vi "1D experiment_v119999.vi"() -> ()   [LabVIEW 2010]
uses:
  ola/Speaker Example/Action Engines/AE Access VIs/AE - Bluetooth Initialise.vi
  ola/Speaker Example/Action Engines/AE Access VIs/AE - Bluetooth Connect All.vi
  <vilib>/Utility/cursorutil.llb/Set Cursor (Cursor ID).vi
  <vilib>/Utility/file.llb/Write To Spreadsheet File (DBL).vi
  User32.dll
panel:
  out "1D Experiment":cluster{"Y":dbl[], "Y":dbl[]}[](graph) caption="Press \"Home\" in WiiMote to STOP"
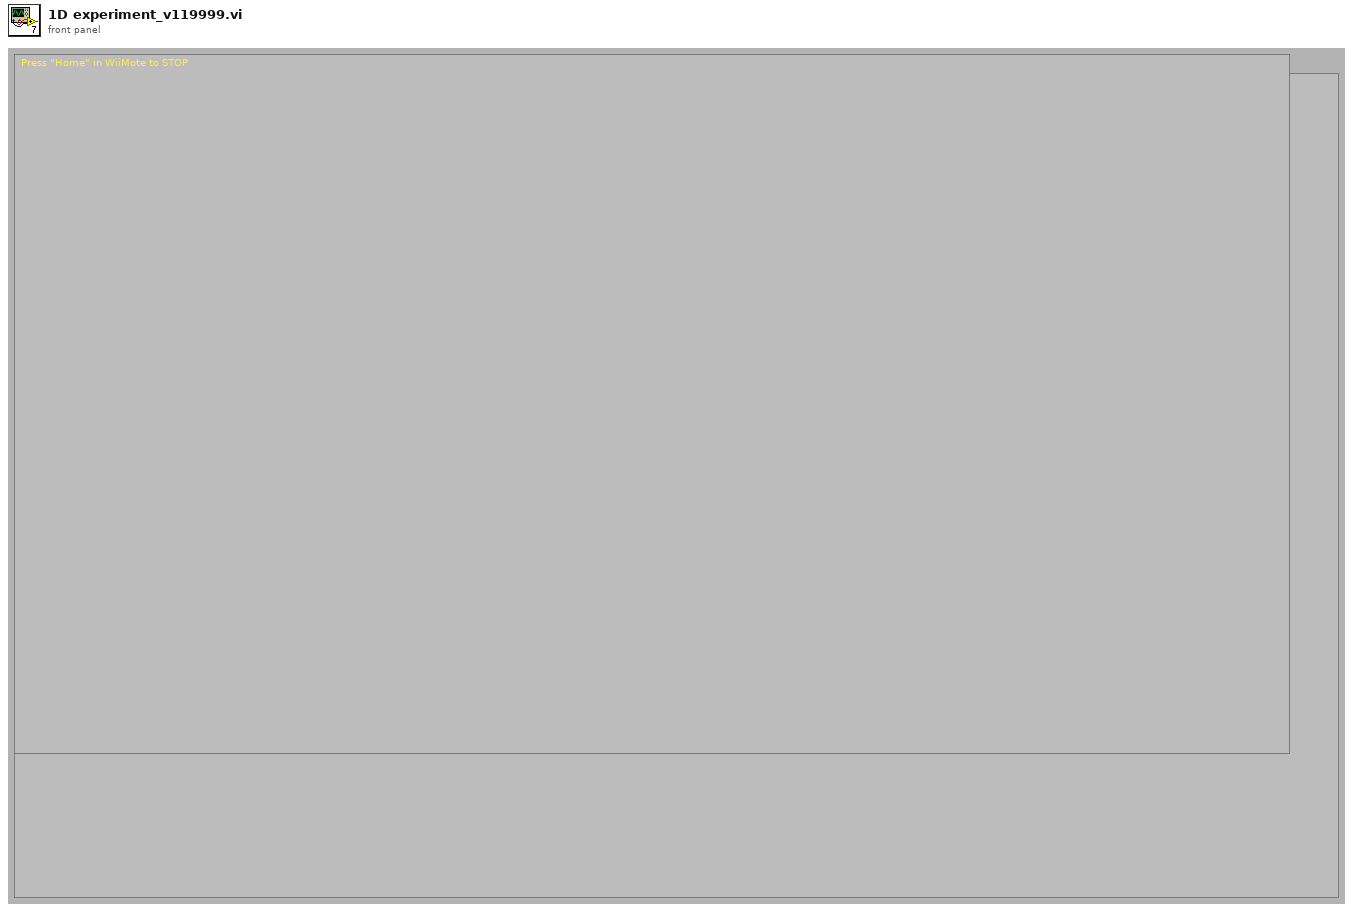
[diagram p1: front panel]
types:
  T1 = enum16{"open", "replace", "create", "open or create", "replace or create", "replace or create with confirmation"}
  T2 = cluster{"Radius":dbl, "Center":dbl, "D":dbl, "Valid":bool}
  T3 = typedef "LVAllMonitorsDisplayTypeDef.ctl" = cluster{"Bounds":cluster{"Left":i16, "Top":i16, "Right":i16, "Bottom":i16}, "Depth":i16}[]
  T4 = cluster{"Bounds":cluster{"Left":i16, "Top":i16, "Right":i16, "Bottom":i16}, "Depth":i16}
  T5 = cluster{"Left":i16, "Top":i16, "Right":i16, "Bottom":i16}
  T6 = typedef "LVPoint32TypeDef.ctl" = cluster{"Horizontal":i32, "Vertical":i32}
  T7 = cluster{"Cursor.Cursor Position:Cursor X":dbl, "Cursor.Cursor Position:Cursor X":dbl}
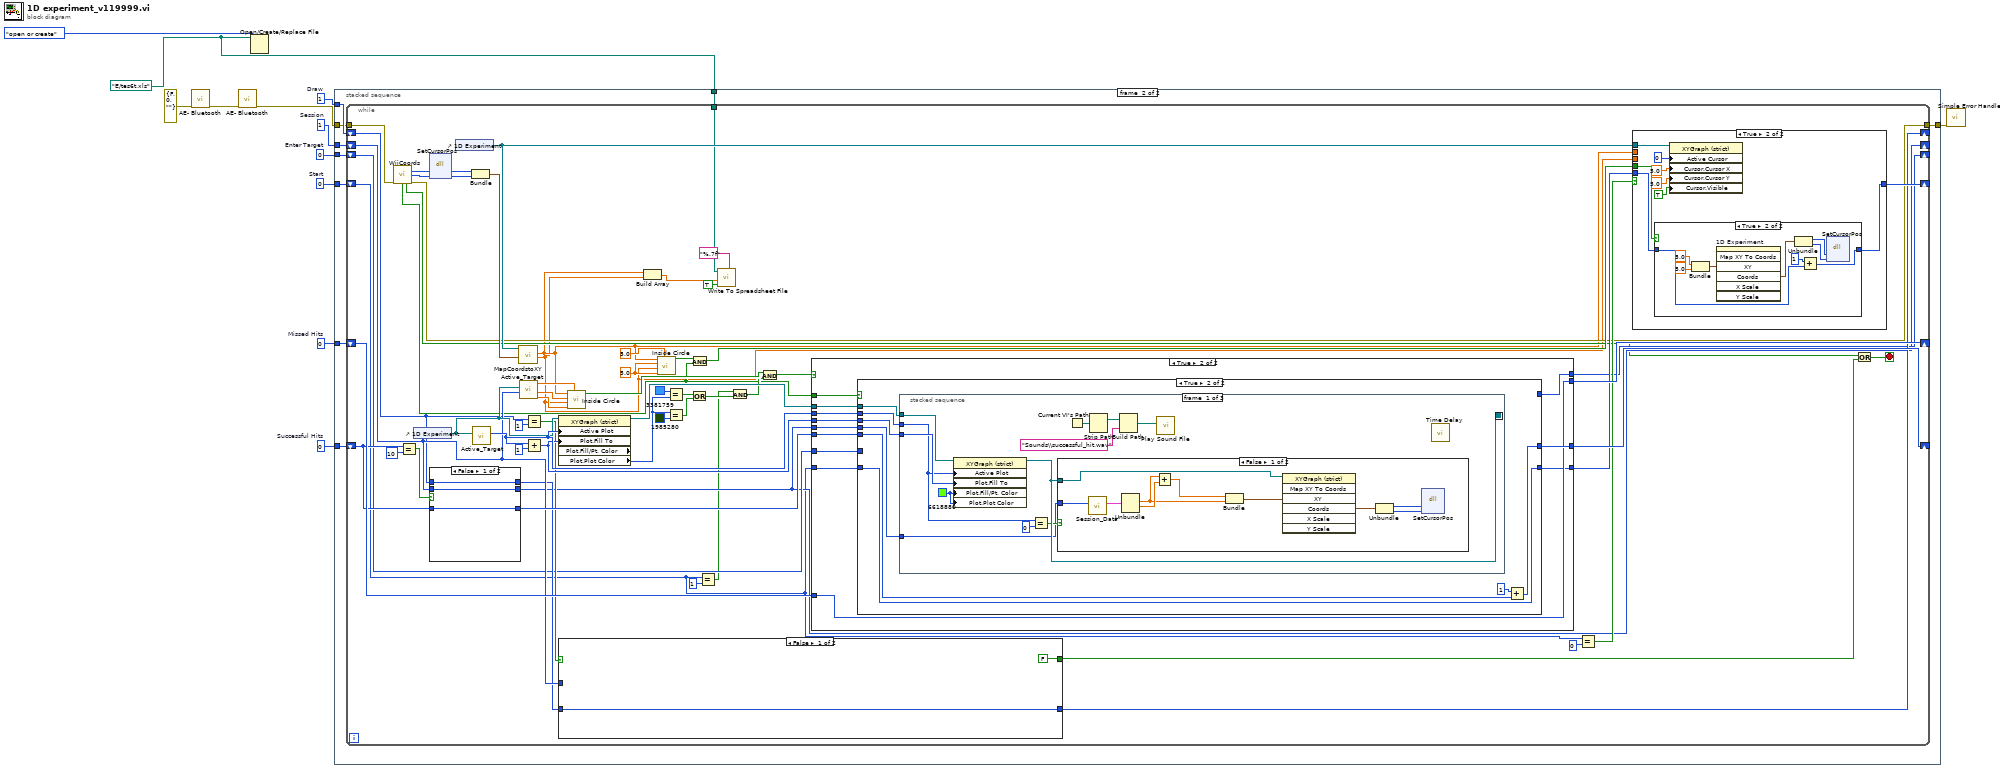
[diagram p0: block diagram]
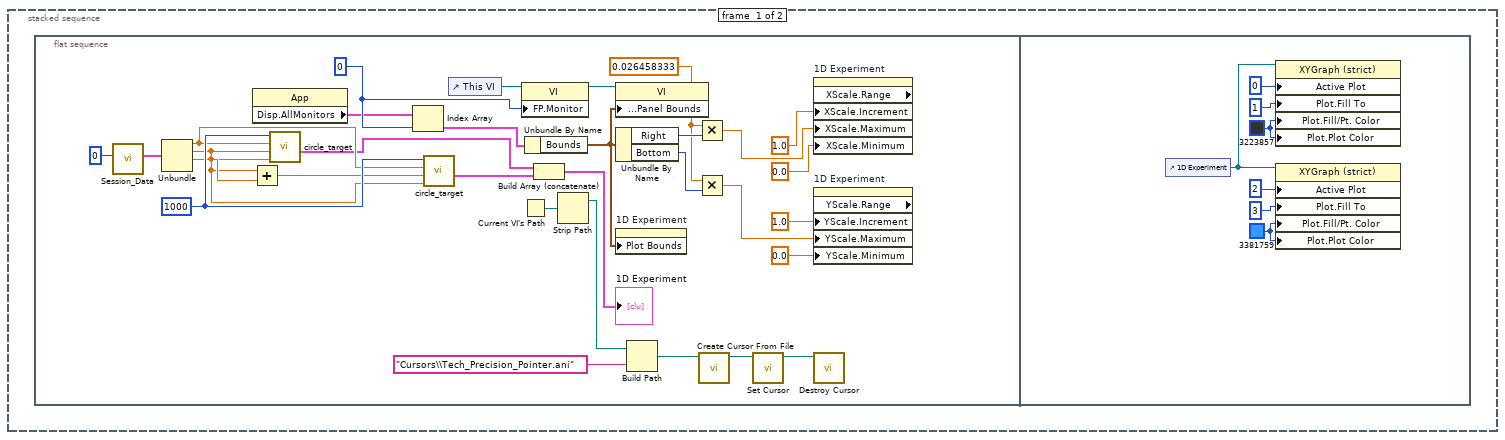
[diagram p2: hidden frame]
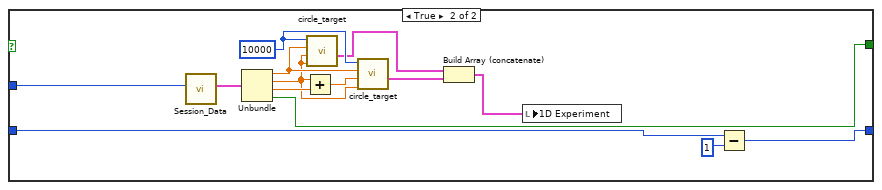
[diagram p3: hidden frame]
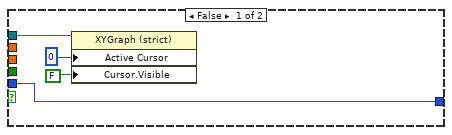
[diagram p4: hidden frame]
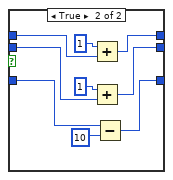
[diagram p6: hidden frame]
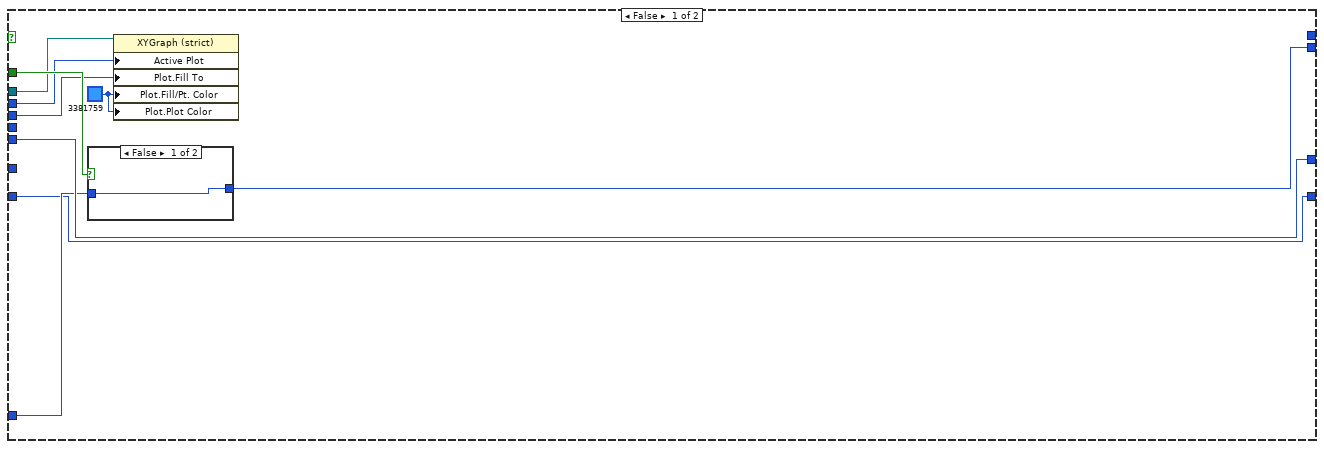
[diagram p7: hidden frame]
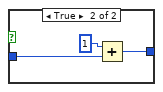
[diagram p8: hidden frame]
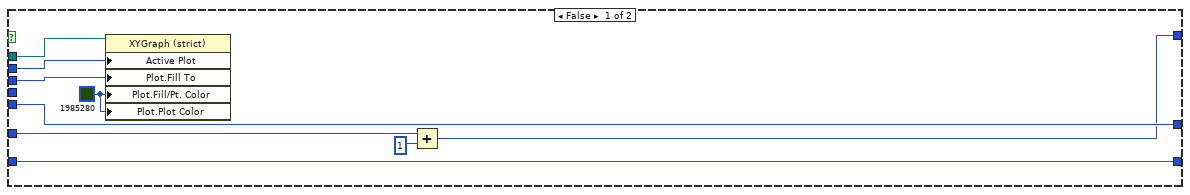
[diagram p9: hidden frame]
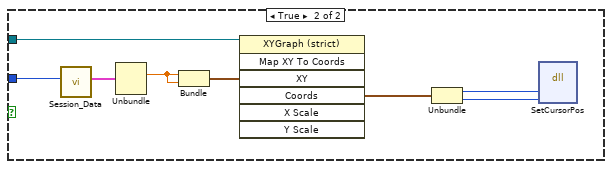
[diagram p10: hidden frame]
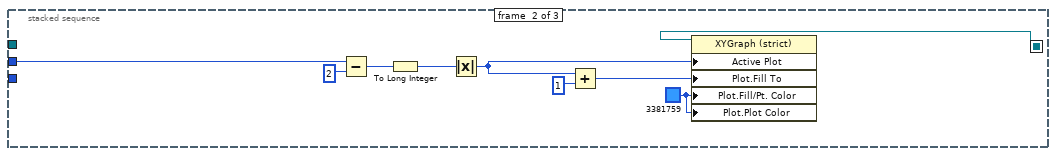
[diagram p11: hidden frame]
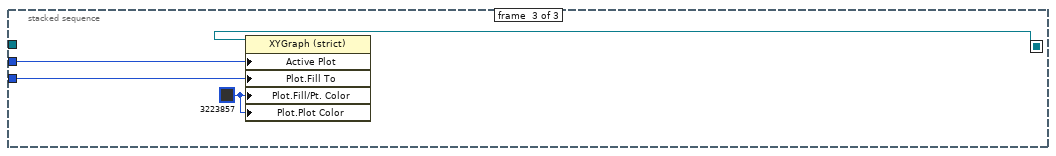
[diagram p12: hidden frame]
diagram:
  w1 = path "E:/tes6t.xls" ("file path (use dialog)")
  w7 = 0  # Enter Target
  w8 = 1  # Draw
  w9 = 0  # Start
  w10 = 1  # Session
  w11 = 0  # Missed Hits
  w12 = 0  # Successful Hits
  n1 = call-poly "AE- Bluetooth.vi"("error in (no error)"=errorcluster {"status"=FALSE, "code"=0, "source"=""}) -> ("error out"=w6:errorcluster)  [unwired: 10 in]
  n2 = call-poly "AE- Bluetooth.vi"("error in (no error)"=w6) -> ("error out"=w4:errorcluster)  [unwired: 9 in, 1 out]
  n3 = Open/Create/Replace File(file path (use dialog)=w1, operation (0:open)=T1."open or create") -> ()  [unwired: 4 in, 3 out]
  n4 = stacked-sequence {
    tunnel: w12 -> [_ w59]
    tunnel: w11 -> [_ w58]
    tunnel: w10 -> [_ w57]
    tunnel: w9 -> [_ w56]
    tunnel: w8 -> [_ w55]
    tunnel: w7 -> [_ w54]
    tunnel: w4 -> [_ w53]
    tunnel: [_ w52] -> w3
    tunnel: w1 -> [_ w51]
    frame #0 {
      n5 = flat-sequence {
        frame #0 {
          w20 = 0.026458333 ("y")
          w31 = u16 0 ("Front Panel Window:Monitor")
          w43 = 1000
          n6 = call "Session_Data.vi"("Session"=0) -> ("output cluster"=w41:T2)  [unwired: 10 in]
          n7 = Unbundle(w41) -> ("Radius"=w40:dbl, "Center"=w38:dbl, "D"=w39:dbl)  [unwired: 1 out]
          n8 = Add(x=w38, y=w39) -> (x+y=w42:dbl)
          n9 = property class="App"() -> ("Disp.AllMonitors"=w30:T3)  [unwired: 2 in, 2 out]
          n10 = call "circle_target.vi"("y0"=w38, "x0"=w38, "Radius"=w40, "Pixels"=w43) -> ("Target plots"=w36:cluster{dbl[], dbl[]}[])  [unwired: 7 in]
          n11 = Index Array(array=w30, index=w31) -> (element=w32:T4)
          n12 = call "circle_target.vi"("y0"=w38, "x0"=w42, "Radius"=w40, "Pixels"=w43) -> ("Target plots"=w37:cluster{dbl[], dbl[]}[])  [unwired: 7 in]
          n13 = control-ref of="This VI"() -> (w33:refnum<vi>)
          n14 = Current VI's Path() -> (path=w28:path)
          n15 = property class="VI"(reference=w33, "FP.Monitor"=w31) -> (reference out=w29:refnum<vi>)  [unwired: 1 in, 1 out]
          n16 = Unbundle By Name(w32) -> ("Bounds"=w22:T5)
          n17 = Build Array (concatenate)(w36, w37) -> (→"1D Experiment":cluster{dbl[], dbl[]}[])
          n18 = Strip Path(path=w28) -> (stripped path=w27:path)  [unwired: 1 out]
          n19 = property class="VI"(reference=w29, "Front Panel Window:Panel Bounds"=w22) -> ()  [unwired: 1 in, 2 out]
          n20 = Unbundle By Name(w22) -> ("Right"=w21:i16, "Bottom"=w19:i16)
          n21 = property on="1D Experiment" class="XYGraph (strict)"("Plot Bounds"=w22) -> ()  [unwired: 2 in, 2 out]
          n22 = Build Path(base path=w27, name or relative path="Cursors\\Tech_Precision_Pointer.ani") -> (appended path=w25:path)
          n23 = Multiply(x=w20, y=w21) -> (x*y=w17:dbl)
          n24 = Multiply(x=w20, y=w19) -> (x*y=w14:dbl)
          n25 = call <vilib>:"Create Cursor From File.vi"("cursor file"=w25) -> ("cursor ID"=w24:refnum<k1>)  [unwired: 9 in, 1 out]
          n26 = call-poly <vilib>:"Set Cursor.vi"("cursor ID"=w24) -> ("previous cursor ID"=w23:refnum<k1>)  [unwired: 9 in, 1 out]
          n27 = property on="1D Experiment" class="XYGraph (strict)" props=["XScale", "Range", "XScale", "Increment", "XScale", "Maximum", "XScale", "Minimum"]("XScale.Increment"=1.0 ("X Scale.Range:Increment"), "XScale.Maximum"=w17, "XScale.Minimum"=0.0 ("X Scale.Range:Minimum")) -> ()  [unwired: 2 in, 3 out]
          n28 = property on="1D Experiment" class="XYGraph (strict)" props=["YScale", "Range", "YScale", "Increment", "YScale", "Maximum", "YScale", "Minimum"]("YScale.Increment"=1.0 ("Y Scale.Range:Increment"), "YScale.Maximum"=w14, "YScale.Minimum"=0.0 ("Y Scale.Range:Minimum")) -> ()  [unwired: 2 in, 3 out]
          n29 = call <vilib>:"Destroy Cursor.vi"("cursor ID"=w23) -> ()  [unwired: 9 in, 1 out]
        }
        frame #1 {
          w49 = u32 3381759
          w46 = u32 3223857
          n30 = control-ref of="1D Experiment"() -> (w50:refnum<vi>)
          n31 = property on="Property Node" class="XYGraph (strict)"(reference=w50, "Active Plot"=u32 0, "Plot.Fill To"=i16 1, "Plot.Fill/Pt. Color"=w46, "Plot.Plot Color"=w46) -> ()  [unwired: 1 in, 2 out]
          n32 = property on="Property Node" class="XYGraph (strict)"(reference=w50, "Active Plot"=u32 2, "Plot.Fill To"=i16 3, "Plot.Fill/Pt. Color"=w49, "Plot.Plot Color"=w49) -> ()  [unwired: 1 in, 2 out]
        }
      }
    }
    frame #1 {
      n33 = while {
        shift-right: [w111] -> _
        shift-left: w59 -> [w92]
        shift-right: [w109] -> _
        shift-left: w58 -> [w110]
        shift-right: [w84] -> _
        shift-left: w57 -> [w93]
        shift-right: [w97] -> _
        shift-left: w56 -> [w83]
        shift-right: [w89] -> _
        shift-left: w55 -> [w90]
        shift-right: [w85] -> _
        shift-left: w54 -> [w86]
        tunnel: w53 -> [w73]
        tunnel: [w66] -> w52
        tunnel: w51 -> [w62]
        stop <- w67 stop-if-true
        w101 = 5.0 ("x0")
        n34 = call "WiiCoords.vi"("error in (no error)"=w73) -> ("X"=w72:i32, "Y"=w70:i32, "A"=w71:bool, "Home"=w68:bool, "error out"=w66:errorcluster)  [unwired: 10 in]
        n35 = Equal?(x=w92, y=10) -> (x = y?=w107:bool)
        n36 = control-ref of="1D Experiment"() -> (w104:refnum<vi>)
        n37 = dll-call lib="User32.dll" fn="SetCursorPos"(w72, w70) -> (w76:i32, w75:i32)  [unwired: 4 in, 2 out]
        n38 = case shown="False" w107 {
          tunnel: w92 -> [w162 w171]
          tunnel: [w162 w169] -> w106
          tunnel: w93 -> [w161 w168]
          tunnel: [w161 w166] -> w84
          tunnel: w90 -> [w160 w165]
          tunnel: [w160 w163] -> w88
          frame False {
          }
          frame True {
            n39 = Add(x=1, y=w165) -> (x+y=w163:i32)
            n40 = Add(x=1, y=w168) -> (x+y=w166:i32)
            n41 = Subtract(x=w171, y=10) -> (x-y=w169:i32)
          }
        }
        n42 = control-ref of="1D Experiment"() -> (w77:refnum<vi>)
        n43 = Bundle(w76, w75) -> (w74:cluster{i32, i32})  [unwired: 1 in]
        n44 = call "Active_Target.vi"("XYGraph Refnum"=w104) -> ("Active Plot"=w115:u32)  [unwired: 7 in, 3 out]
        n45 = call "MapCoordstoXY.vi"("Coordinates"=w74, "XYGraph Refnum"=w77) -> ("Y(graph)"=w64:dbl, "X (graph)"=w65:dbl)  [unwired: 7 in]
        n46 = call "Active_Target.vi"("Session"=w93, "XYGraph Refnum"=w104) -> ("y0"=w112:dbl, "x0"=w113:dbl, "Radius"=w105:dbl)  [unwired: 6 in, 1 out]
        n47 = Equal?(x=w90, y=1) -> (x = y?=w87:bool)
        n48 = Add(x=w115, y=u32 1) -> (x+y=w114:u32)
        n49 = property on="Property Node" class="XYGraph (strict)" props=["Active Plot", "Plot", "Fill To", "Plot", "Fill/Pt. Color", "Plot", "Plot Color"](reference=w104, "Active Plot"=w115, "Plot.Fill To"=w114) -> (reference out=w94:refnum<vi>, "Plot.Plot Color"=w96:u32)  [unwired: 1 in, 2 out]
        n50 = case shown="False" w87 {
          tunnel: [FALSE ("Valid") w129] -> w69
          tunnel: w93 -> [_ w128]
          tunnel: [w122 w126] -> w89
          tunnel: w88 -> [w122 w125]
          frame False {
          }
          frame True {
            w137 = 10000
            n51 = call "Session_Data.vi"("Session"=w128) -> ("output cluster"=w135:T2)  [unwired: 10 in]
            n52 = Unbundle(w135) -> ("Radius"=w134:dbl, "Center"=w132:dbl, "D"=w133:dbl, "Valid"=w129:bool)
            n53 = Add(x=w132, y=w133) -> (x+y=w136:dbl)
            n54 = call "circle_target.vi"("y0"=w132, "x0"=w132, "Radius"=w134, "Pixels"=w137) -> ("Target plots"=w131:cluster{dbl[], dbl[]}[])  [unwired: 7 in]
            n55 = call "circle_target.vi"("y0"=w132, "x0"=w136, "Radius"=w134, "Pixels"=w137) -> ("Target plots"=w130:cluster{dbl[], dbl[]}[])  [unwired: 7 in]
            n56 = Build Array (concatenate)(w131, w130) -> (w124:cluster{dbl[], dbl[]}[])
            n57 = local write "1D Experiment"(w124) -> ()
            n58 = Subtract(x=w125, y=1) -> (x-y=w126:i32)
          }
        }
        n59 = call "Inside Circle.vi"("Radius"=w105, "y0"=w112, "y"=w64, "x0"=w113, "x"=w65) -> ("Inside Circle"=w80:bool)  [unwired: 6 in]
        n60 = Build Array(w65, w64) -> (w63:dbl[])
        n61 = call "Inside Circle.vi"("Radius"=5.0, "y0"=w101, "y"=w64, "x0"=w101, "x"=w65) -> ("Inside Circle"=w99:bool)  [unwired: 6 in]
        n62 = Equal?(x=u32 3381759, y=w96) -> (x = y?=w118:bool)
        n63 = Equal?(x=w96, y=u32 1985280) -> (x = y?=w117:bool)
        n64 = Or(x=w118, y=w117) -> (x .or. y?=w81:bool)
        n65 = And(x=w99, y=w71) -> (x .and. y?=w98:bool)
        n66 = Equal?(x=w83, y=1) -> (x = y?=w79:bool)
        n67 = call-poly <vilib>:"Write To Spreadsheet File.vi"("format (%.3f)"="%.7f", "append to file? (new file:F)"=TRUE, "1D data"=w63, "file path (dialog if empty)"=w62) -> ()  [unwired: 4 in, 1 out]
        n68 = And(x=w79, y=w81) -> (x .and. y?=w78:bool)
        n69 = And(x=w80, y=w78) -> (x .and. y?=w120:bool)
        n70 = case shown="True" w120 {
          tunnel: w71 -> [w178 w196]
          tunnel: w115 -> [w175 w192]
          tunnel: w114 -> [w174 w191]
          tunnel: w106 -> [w179 w195]
          tunnel: [w179 w194] -> w111
          tunnel: w110 -> [w177 w193]
          tunnel: [w176 w193] -> w109
          tunnel: w83 -> [w173 w190]
          tunnel: [w173 w189] -> w95
          tunnel: w94 -> [w172 w188]
          tunnel: w86 -> [_ w187]
          tunnel: [_ w186] -> w85
          tunnel: w84 -> [_ w185]
          frame False {
            w180 = u32 3381759
            n71 = case shown="False" w178 {
              tunnel: w177 -> [w181 w184]
              tunnel: [w181 w182] -> w176
              frame False {
              }
              frame True {
                n72 = Add(x=1, y=w184) -> (x+y=w182:i32)
              }
            }
            n73 = property on="Property Node" class="XYGraph (strict)"(reference=w172, "Active Plot"=w175, "Plot.Fill To"=w174, "Plot.Fill/Pt. Color"=w180, "Plot.Plot Color"=w180) -> ()  [unwired: 1 in, 2 out]
          }
          frame True {
            n74 = case shown="True" w196 {
              tunnel: w195 -> [w204 w213]
              tunnel: [w204 w207] -> w194
              tunnel: w192 -> [w203 w211]
              tunnel: w191 -> [w202 w210]
              tunnel: w190 -> [w201 w209]
              tunnel: [w201 w209] -> w189
              tunnel: w188 -> [w200 w208]
              tunnel: w187 -> [w199 _]
              tunnel: [w197 _] -> w186
              tunnel: w185 -> [_ w206]
              frame False {
                w205 = u32 1985280
                n75 = property on="Property Node" class="XYGraph (strict)"(reference=w200, "Active Plot"=w203, "Plot.Fill To"=w202, "Plot.Fill/Pt. Color"=w205, "Plot.Plot Color"=w205) -> ()  [unwired: 1 in, 2 out]
                n76 = Add(x=w199, y=1) -> (x+y=w197:i32)
              }
              frame True {
                n77 = stacked-sequence {
                  seq-local: [w222 _ _] -> [_ w244 w253]
                  tunnel: w211 -> [w221 w245 w255]
                  tunnel: w210 -> [w224 _ w254]
                  tunnel: w208 -> [w223 _ _]
                  tunnel: w206 -> [w218 _ _]
                  frame #0 {
                    w225 = u32 6618880
                    n78 = property on="Property Node" class="XYGraph (strict)"(reference=w223, "Active Plot"=w221, "Plot.Fill To"=w224, "Plot.Fill/Pt. Color"=w225, "Plot.Plot Color"=w225) -> (reference out=w222:refnum<vi>)  [unwired: 1 in, 1 out]
                    n79 = Equal?(x=w221, y=u32 0) -> (x = y?=w219:bool)
                    n80 = case shown="False" w219 {
                      tunnel: w222 -> [w231 w236]
                      tunnel: w218 -> [w228 w240]
                      frame False {
                        n81 = call "Session_Data.vi"("Session"=w228) -> ("output cluster"=w232:T2)  [unwired: 10 in]
                        n82 = Unbundle(w232) -> ("Center"=w226:dbl, "D"=w230:dbl)  [unwired: 2 out]
                        n83 = Add(x=w226, y=w230) -> (x+y=w227:dbl)
                        n84 = Bundle(w227, "Center"=w226) -> (w229:cluster{dbl, "Center":dbl})  [unwired: 1 in]
                        n85 = invoke on="Invoke Node" class="XYGraph (strict)" method="Map XY To Coords"(reference=w231, "XY"=w229) -> ("Coords"=w235:T6)  [unwired: 5 in, 6 out]
                        n86 = Unbundle(w235) -> ("Horizontal"=w234:i32, "Vertical"=w233:i32)
                        n87 = dll-call lib="User32.dll" fn="SetCursorPos"(w234, w233) -> ()  [unwired: 6 in, 2 out]
                      }
                      frame True {
                        n88 = call "Session_Data.vi"("Session"=w240) -> ("output cluster"=w239:T2)  [unwired: 10 in]
                        n89 = Unbundle(w239) -> ("Center"=w238:dbl)  [unwired: 3 out]
                        n90 = Bundle("Center"=w238, "Center"=w238) -> (w237:cluster{"Center":dbl, "Center":dbl})  [unwired: 1 in]
                        n91 = invoke on="Invoke Node" class="XYGraph (strict)" method="Map XY To Coords"(reference=w236, "XY"=w237) -> ("Coords"=w243:T6)  [unwired: 5 in, 6 out]
                        n92 = Unbundle(w243) -> ("Horizontal"=w242:i32, "Vertical"=w241:i32)
                        n93 = dll-call lib="User32.dll" fn="SetCursorPos"(w242, w241) -> ()  [unwired: 6 in, 2 out]
                      }
                    }
                    n94 = Current VI's Path() -> (path=w215:path)
                    n95 = Strip Path(path=w215) -> (stripped path=w214:path)  [unwired: 1 out]
                    n96 = Build Path(base path=w214, name or relative path="Sounds\\successful_hit.wav") -> (appended path=w216:path)
                    n97 = call <vilib>:"Play Sound File.vi"("path"=w216) -> ()  [unwired: 9 in, 2 out]
                    n98 = call "Time Delay"() -> ()  [unwired: 11 in, 1 out]
                  }
                  frame #1 {
                    w252 = u32 3381759
                    n99 = Subtract(x=w245, y=u32 2) -> (x-y=w249:u32)
                    n100 = To Long Integer(number=w249) -> (32bit integer=w248:i32)
                    n101 = Absolute Value(x=w248) -> (abs(x)=w246:i32)
                    n102 = Add(x=w246, y=u32 1) -> (x+y=w250:u32)
                    n103 = property on="Property Node" class="XYGraph (strict)"(reference=w244, "Active Plot"=w246, "Plot.Fill To"=w250, "Plot.Fill/Pt. Color"=w252, "Plot.Plot Color"=w252) -> ()  [unwired: 1 in, 2 out]
                  }
                  frame #2 {
                    w256 = u32 3223857
                    n104 = property on="Property Node" class="XYGraph (strict)"(reference=w253, "Active Plot"=w255, "Plot.Fill To"=w254, "Plot.Fill/Pt. Color"=w256, "Plot.Plot Color"=w256) -> ()  [unwired: 1 in, 2 out]
                  }
                }
                n105 = Add(x=1, y=w213) -> (x+y=w207:i32)
              }
            }
          }
        }
        n106 = Equal?(x=w83, y=0) -> (x = y?=w102:bool)
        n107 = case shown="True" w102 {
          tunnel: w77 -> [w138 w143]
          tunnel: w65 -> [_ _]
          tunnel: w64 -> [_ _]
          tunnel: w98 -> [_ w146]
          tunnel: w95 -> [w141 w145]
          tunnel: [w141 w144] -> w97
          frame False {
            n108 = property on="Property Node" class="XYGraph (strict)"(reference=w138, "Active Cursor"=u32 0, "Cursor.Visible"=FALSE) -> ()  [unwired: 1 in, 2 out]
          }
          frame True {
            n109 = case shown="True" w146 {
              tunnel: w145 -> [w150 w159]
              tunnel: [w150 w157] -> w144
              frame False {
              }
              frame True {
                n110 = Bundle("Cursor.Cursor Position:Cursor X"=5.0, "Cursor.Cursor Position:Cursor X"=5.0) -> (w154:T7)  [unwired: 1 in]
                n111 = invoke on="1D Experiment" class="XYGraph (strict)" method="Map XY To Coords"("XY"=w154) -> ("Coords"=w153:T6)  [unwired: 6 in, 6 out]
                n112 = Unbundle(w153) -> ("Horizontal"=w152:i32, "Vertical"=w151:i32)
                n113 = Add(x=1, y=w159) -> (x+y=w157:i32)
                n114 = dll-call lib="User32.dll" fn="SetCursorPos"(w152, w151) -> ()  [unwired: 6 in, 2 out]
              }
            }
            n115 = property on="Property Node" class="XYGraph (strict)"(reference=w143, "Active Cursor"=u32 0, "Cursor.Cursor X"=5.0 ("Cursor.Cursor Position:Cursor X"), "Cursor.Cursor Y"=5.0 ("Cursor.Cursor Position:Cursor Y"), "Cursor.Visible"=TRUE) -> ()  [unwired: 1 in, 2 out]
          }
        }
        n116 = Or(x=w68, y=w69) -> (x .or. y?=w67:bool)
      }
    }
  }
  n117 = call <vilib>:"Simple Error Handler.vi"("error in (no error)"=w3) -> ()  [unwired: 4 in, 5 out]
